vi "source absorption.vi"(7 "python in":refnum<k35>, 8 "error in":errorcluster, 11 "Source In":dbl[][](array[numeric])) -> (0 "error out":errorcluster, 3 "Source Out":dbl[][](array[numeric]), 5 "python out":refnum<k35>)   [LabVIEW 2023]
uses:
  <vilib>/Utility/file.llb/Read Delimited Spreadsheet (string).vi
panel:
  out "Cs Total":dbl
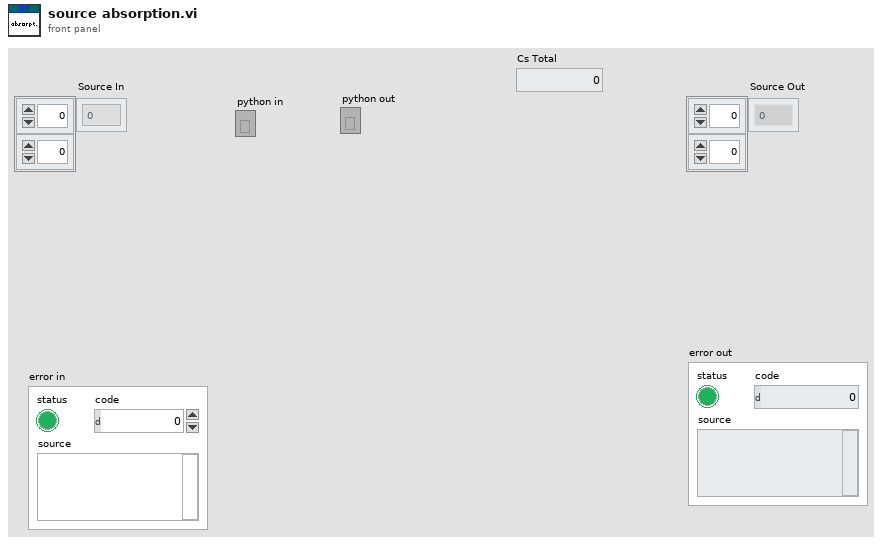
[diagram p1: front panel]
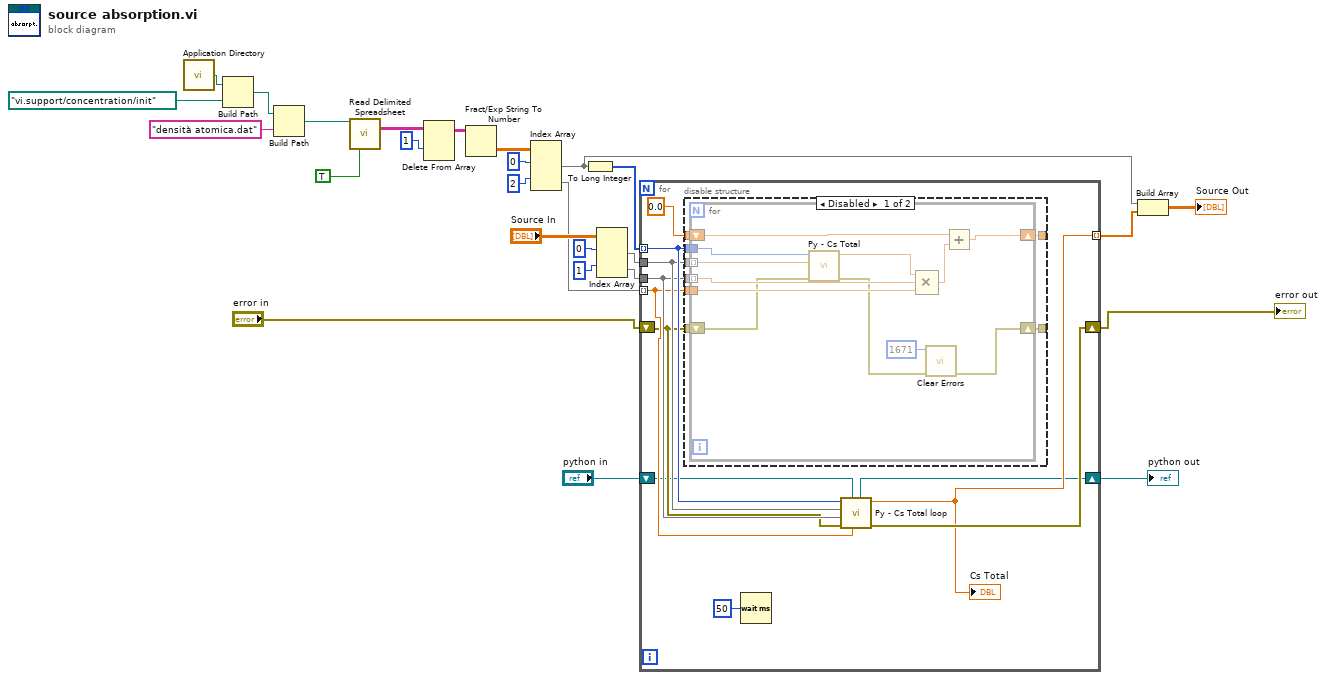
[diagram p0: block diagram]
diagram:
  n1 = call <vilib>:"Application Directory.vi"() -> ("Application Directory"=w24:path)
  n2 = Build Path(base path=w24, name or relative path=path "vi.support/concentration/init") -> (appended path=w21:path)
  n3 = Build Path(base path=w21, name or relative path="densità atomica.dat") -> (appended path=w19:path)
  n4 = call-poly <vilib>:"Read Delimited Spreadsheet.vi"("file path (dialog if empty)"=w19, "transpose? (F)"=TRUE) -> ("all rows"=w17:string[][])  [unwired: 8 in, 5 out]
  n5 = Delete From Array(array=w17, index (row)=1) -> (array with subset deleted=w16:string[][])  [unwired: 2 in, 1 out]
  n6 = Fract/Exp String To Number(string=w16) -> (number=w13:dbl[][])  [unwired: 3 in, 1 out]
  n7 = Index Array(array=w13, index (row) #1=0 ("index (row)"), index (row) #2=2 ("index (row)")) -> (element #1=w6:dbl[], element #2=w11:dbl[])  [unwired: 2 in]
  n8 = To Long Integer(number=w6) -> (32bit integer=w8:i32[])
  n9 = Index Array(array="Source In", index (row) #1=0 ("index (row)"), index (row) #2=1 ("index (row)")) -> (element #1=w10:dbl[], element #2=w9:dbl[])  [unwired: 2 in]
  n10 = for {
    tunnel: w11 -> [w33] mode=indexing
    tunnel: w10 -> [w35]
    tunnel: w9 -> [w34]
    tunnel: [w30] -> w7 mode=indexing
    tunnel: w8 -> [w36] mode=indexing
    shift-right: [w31] -> w4
    shift-left: "error in" -> [w32]
    shift-right: [w28] -> w1
    shift-left: "python in" -> [w29]
    n11 = disable-structure shown="Disabled" {
      disable-tunnel: 0.0 -> [w45 _]
      disable-tunnel: [w44 _] -> _
      disable-tunnel: w32 -> [w43 _]
      disable-tunnel: [w42 _] -> _
      disable-tunnel: w36 -> [w41 _]
      disable-tunnel: w35 -> [w40 _]
      disable-tunnel: w34 -> [w39 _]
      disable-tunnel: w33 -> [w38 _]
      frame Disabled {
        n12 = for {
          tunnel: w40 -> [w51] mode=indexing
          tunnel: w38 -> [w56]
          tunnel: w39 -> [w57] mode=indexing
          shift-right: [w54] -> w44
          shift-left: w45 -> [w53]
          tunnel: w41 -> [w52]
          shift-right: [w46] -> w42
          shift-left: w43 -> [w50]
          n13 = call "Py - Cs Total.vi"("error in"=w50, "En"=w51, "Z"=w52) -> ("error out"=w47:errorcluster, "Cs Total"=w49:dbl)  [unwired: 7 in]
          n14 = Compound Arithmetic op=MULTIPLY(w49, w57, w56) -> (w55:dbl)
          n15 = call <vilib>:"Clear Errors.vi"("error in (no error)"=w47, "specific error code to clear (0: all)"=1671) -> ("error out"=w46:errorcluster)  [unwired: 4 in, 1 out]
          n16 = Add(x=w53, y=w55) -> (x+y=w54:dbl)
        }
      }
      frame Enabled {
      }
    }
    n17 = Wait (ms)(milliseconds to wait=u32 50) -> ()  [unwired: 1 out]
    n18 = call "Py - Cs Total loop.vi"("rho"=w33, "python in"=w29, "error in"=w32, "Int_array"=w34, "En_array"=w35, "Z"=w36) -> ("error out"=w31:errorcluster, "Cs Total"=w30:dbl, "python out"=w28:refnum<k35>)  [unwired: 3 in]
    "Cs Total" <- w30
  }
  "error out" <- w4
  "python out" <- w1
  n19 = Build Array(w6, w7) -> (→"Source Out":dbl[][])
